vi "HEXAA 1.vi"() -> ()   [LabVIEW 2020]
panel:
  out "Waveform Chart":dbl(graph)
  in  "Ok":bool
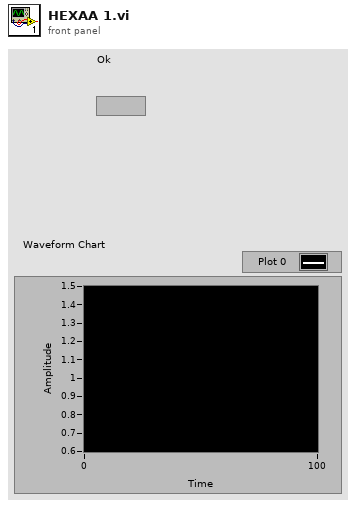
[diagram p1: front panel]
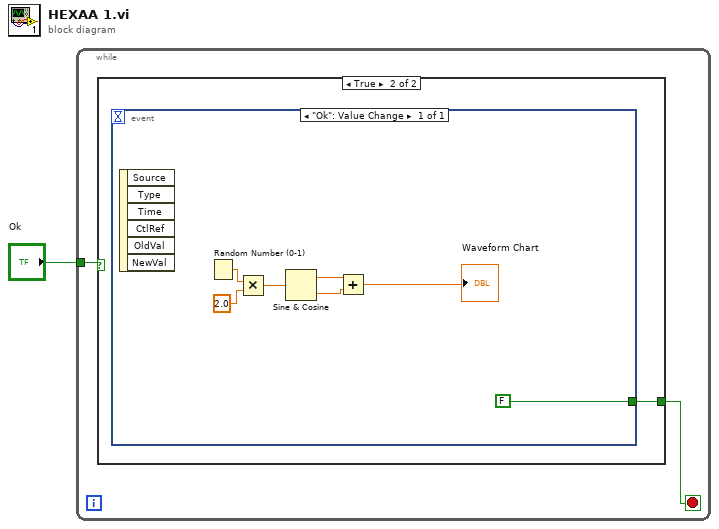
[diagram p0: block diagram]
diagram:
  n1 = while {
    tunnel: "Ok" -> [w2]
    stop <- w3 stop-if-true
    n2 = case shown="True" w2 {
      tunnel: [_ w4] -> w3
      frame False {
      }
      frame True {
        n3 = event shown="[0] \"Ok\": Value Change" {
          selector: _ -> [_]
          dyn-events: _ -> [_]
          timeout: _ -> [_]
          tunnel: [FALSE] -> w4
          event "Ok": Value Change {
            n4 = event-data() -> ()  [unwired: 1 in, 6 out]
            n5 = Random Number (0-1)() -> (number: 0 to 1=w11:dbl)
            n6 = Multiply(x=w11, y=2.0) -> (x*y=w9:dbl)
            n7 = Sine & Cosine(0:w9) -> (1:w7:dbl, 2:w8:dbl)
            n8 = Add(x=w7, y=w8) -> (x+y=→"Waveform Chart":dbl)
          }
        }
      }
    }
  }
